vi "FormatTreeStyle.vi"(7 "Format Command":T1, 8 "Error In":errorcluster, 9 "Row Index":i32, 11 "Tree Refnum":refnum<vi>) -> (0 "Error Out":errorcluster)   [LabVIEW 2012]
doc: "This VI implements the formatting of table data which includes highlighting, unhighlighting, and modifying visible rows (due to scrolling).\n\n<b>INPUTS</b>\n--------\n<b>Format Command </b> - Formatting action needs to be be taken\n<b>Table references array </b>- Array containing references of the tables of interest\n<b>Row </b>- Row number that needs to be fromatted"
uses:
  FormatTree&TableStyle_Commands.ctl
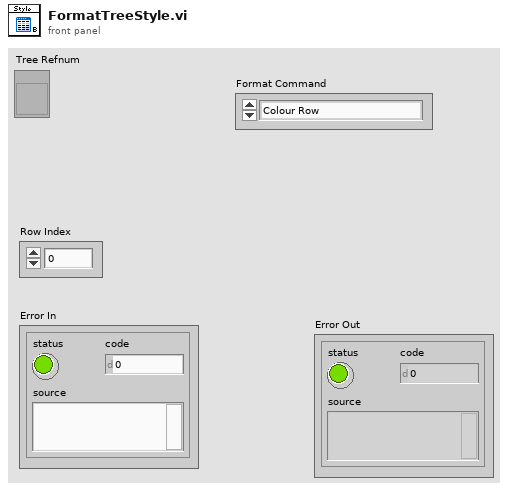
[diagram p1: front panel]
types:
  T1 = typedef "FormatTree&TableStyle_Commands.ctl" = enum16{"Colour Row", "Uncolour Row", "Bold Row", "Unbold Row", "Clear", "UpdateVisibleRows"}
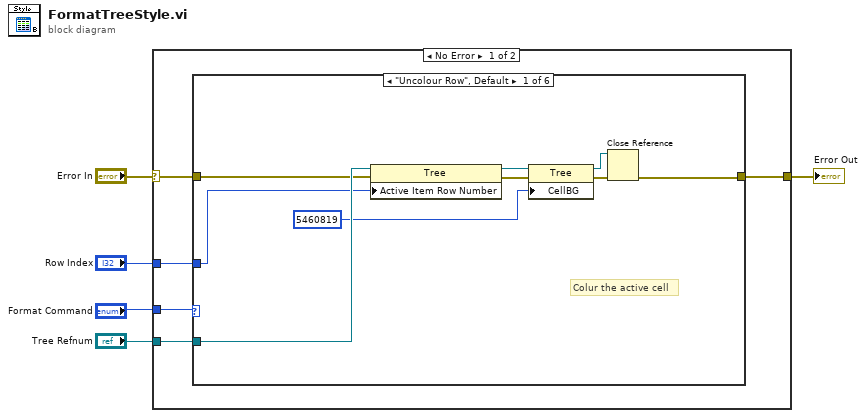
[diagram p0: block diagram]
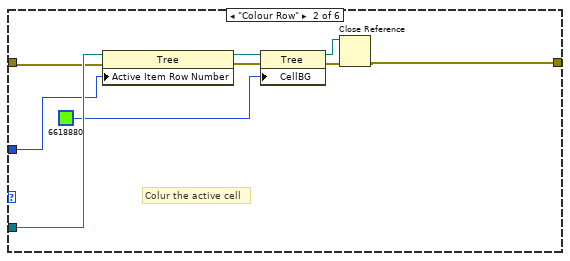
[diagram p2: hidden frame]
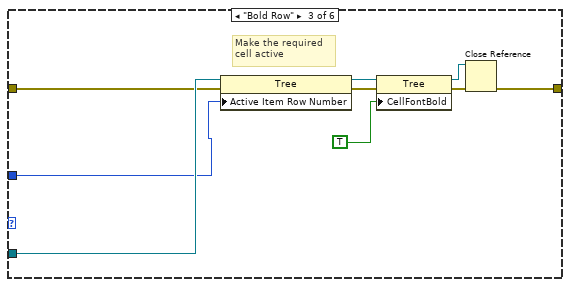
[diagram p3: hidden frame]
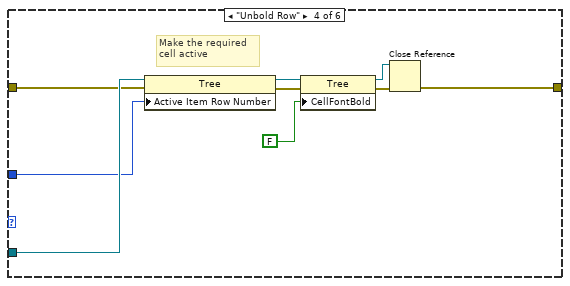
[diagram p4: hidden frame]
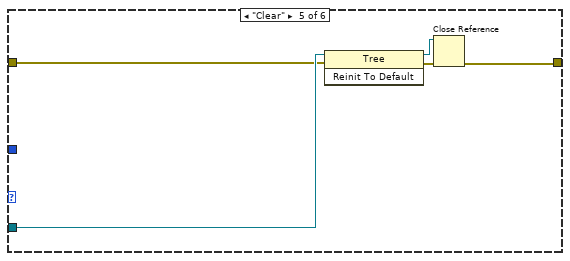
[diagram p5: hidden frame]
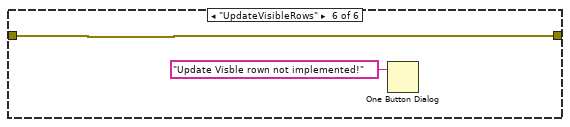
[diagram p6: hidden frame]
diagram:
  n1 = case shown="No Error" "Error In" {
    selector: "Error In" -> [w10 w54]
    tunnel: "Row Index" -> [w9 _]
    tunnel: [w8 w54] -> w3
    tunnel: "Format Command" -> [w7 _]
    tunnel: "Tree Refnum" -> [w6 _]
    frame No Error {
      n2 = case shown="\"Uncolour Row\", Default" w7 {
        tunnel: w10 -> [w12 w20 w29 w39 w47 w53]
        tunnel: w9 -> [w18 w23 w32 w38 _ _]
        tunnel: [w13 w22 w31 w41 w48 w53] -> w8
        tunnel: w6 -> [w19 w24 w33 w42 w51 _]
        frame "Uncolour Row", Default {
          # "Colur the active cell"
          n3 = property class="Tree"(reference=w19, error in=w12, "Active Item Row Number"=w18) -> (reference out=w16:refnum<vi>, error out=w17:errorcluster)
          n4 = property class="Tree"(reference=w16, error in=w17, "CellBG"=u32 5460819 ("Active Cell:Cell Background Color")) -> (reference out=w14:refnum<vi>, error out=w15:errorcluster)
          n5 = Close Reference(reference=w14, error in (no error)=w15) -> (error out=w13:errorcluster)
        }
        frame "Colour Row" {
          # "Colur the active cell"
          n6 = property class="Tree"(reference=w24, error in=w20, "Active Item Row Number"=w23) -> (reference out=w27:refnum<vi>, error out=w28:errorcluster)
          n7 = property class="Tree"(reference=w27, error in=w28, "CellBG"=u32 6618880 ("Background colour")) -> (reference out=w25:refnum<vi>, error out=w26:errorcluster)
          n8 = Close Reference(reference=w25, error in (no error)=w26) -> (error out=w22:errorcluster)
        }
        frame "Bold Row" {
          # "Make the required cell active"
          n9 = property class="Tree"(reference=w33, error in=w29, "Active Item Row Number"=w32) -> (reference out=w36:refnum<vi>, error out=w37:errorcluster)
          n10 = property class="Tree"(reference=w36, error in=w37, "CellFontBold"=TRUE ("Active Cell:Cell Font:Bold")) -> (reference out=w34:refnum<vi>, error out=w35:errorcluster)
          n11 = Close Reference(reference=w34, error in (no error)=w35) -> (error out=w31:errorcluster)
        }
        frame "Unbold Row" {
          # "Make the required cell active"
          n12 = property class="Tree"(reference=w42, error in=w39, "Active Item Row Number"=w38) -> (reference out=w45:refnum<vi>, error out=w46:errorcluster)
          n13 = property class="Tree"(reference=w45, error in=w46, "CellFontBold"=FALSE ("Active Cell:Cell Font:Bold")) -> (reference out=w43:refnum<vi>, error out=w44:errorcluster)
          n14 = Close Reference(reference=w43, error in (no error)=w44) -> (error out=w41:errorcluster)
        }
        frame "Clear" {
          n15 = invoke class="Tree" method="Reinit To Default"(reference=w51, error in=w47) -> (reference out=w49:refnum<vi>, error out=w50:errorcluster)  [unwired: 1 in, 1 out]
          n16 = Close Reference(reference=w49, error in (no error)=w50) -> (error out=w48:errorcluster)
        }
        frame "UpdateVisibleRows" {
          n17 = One Button Dialog(message="Update Visble rown not implemented!") -> ()  [unwired: 1 in, 1 out]
        }
      }
    }
    frame Error {
    }
  }
  "Error Out" <- w3
